vi "Main.vi"(8 "error in (no error)":errorcluster, 11 "InterfaceView in":refnum<class "InterfaceView.lvclass">) -> (0 "error out":errorcluster, 3 "InterfaceView out":refnum<class "InterfaceView.lvclass">)   [LabVIEW 2020, in "Container.lvlib" / "InterfaceView.lvclass"]
uses:
  InterfaceView.lvclass
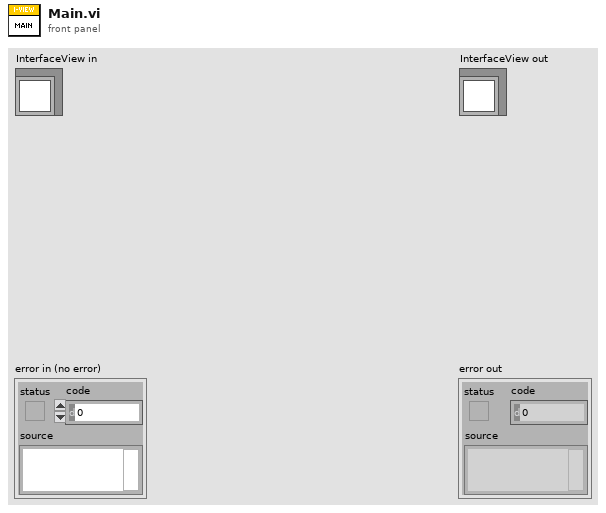
[diagram p1: front panel]
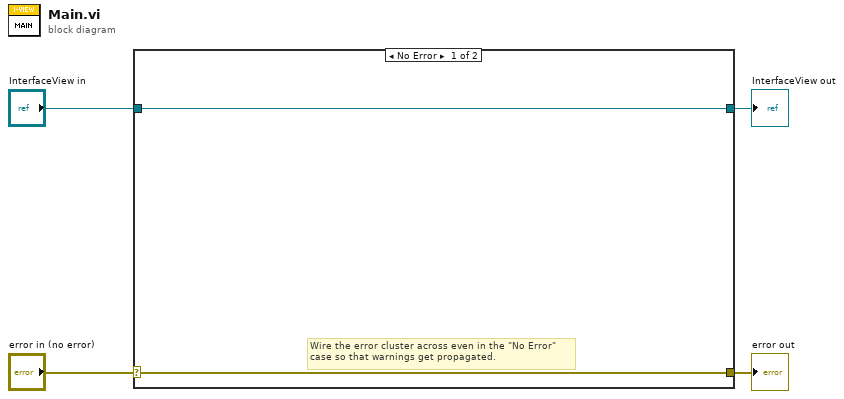
[diagram p0: block diagram]
diagram:
  n1 = case shown="No Error" "error in (no error)" {
    selector: "error in (no error)" -> [w5 w8]
    tunnel: [w5 w8] -> w3
    tunnel: [w6 w7] -> w1
    tunnel: "InterfaceView in" -> [w6 w7]
    frame No Error {
      # "Wire the error cluster across even in the \"No Error\"\ncase so that warnings get propagated."
    }
    frame Error {
    }
  }
  "error out" <- w3
  "InterfaceView out" <- w1
